vi "Configure Humidifiers.vi"(8 "error in":errorcluster, 10 "Humidifier":string="Med", 11 "Controller in":refnum<class "Controller.lvclass">) -> (0 "error out":errorcluster, 1 "TEC Handle":string, 2 "Vaisala Handle":string, 3 "Controller Out":refnum<class "Controller.lvclass">, 5 "MFC":string)   [LabVIEW 2014, in "Controller.lvlib" / "Controller.lvclass"]
uses:
  Controller.lvclass
  reusable/Session APIs/File Access/Config Data/Config Data.lvclass
  <vilib>/Utility/config.llb/NI_LVConfig.lvlib
  <vilib>/Utility/config.llb/Read Key (String).vi
  <vilib>/Utility/config.llb/Read Key (Double).vi
  reusable/Session APIs/CVT/CVT.lvclass
  <vilib>/Utility/config.llb/Read Key (Boolean).vi
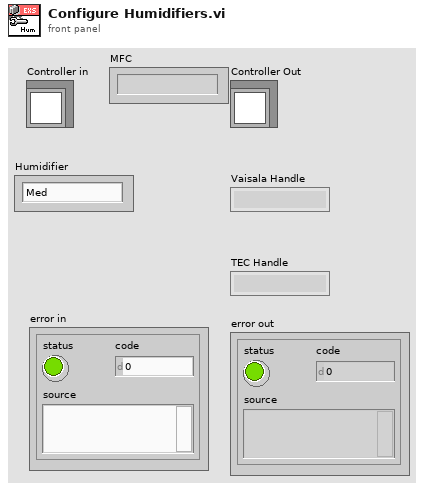
[diagram p1: front panel]
types:
  T1 = typedef "Session - Root.lvclass/Session Handle.ctl" = refnum<data-value>
  T2 = typedef "NI_LVConfig.lvlib/Config Data RefNum.ctl" = refnum<k1>
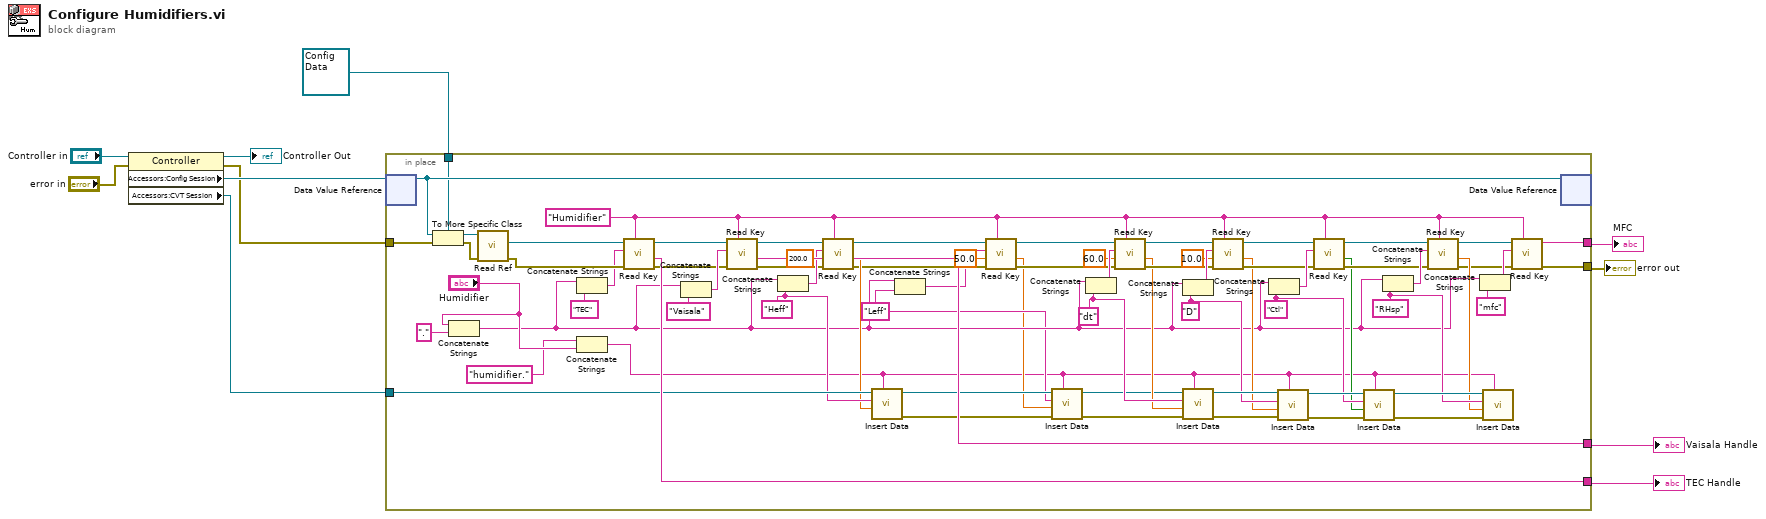
[diagram p0: block diagram]
diagram:
  n1 = property class="Controller"(reference="Controller in", error in="error in") -> (reference out=→"Controller Out":refnum<class "Controller.lvclass">, error out=w3:errorcluster, "Accessors:Config Session"=w7:T1, "Accessors:CVT Session"=w6:T1)
  n2 = in-place {
    in-place-border: refnum<class "Config Data.lvclass"> refnum ("Config Data in") -> [w81]
    in-place-border: [w79] -> w10
    in-place-border: [w78] -> w11
    in-place-border: w3 -> [w76]
    in-place-border: w6 -> [w75]
    in-place-border: [w31] -> w2
    in-place-border: [w29] -> w1
    w18 = "Leff" ("string")
    w39 = "RHsp" ("string")
    w43 = "Ctl" ("string")
    w47 = "D" ("string")
    w51 = "dt" ("string")
    w53 = "Heff" ("string")
    w21 = "Humidifier" ("section")
    n3 = in-place-dvr #1(w7) -> (w82:refnum<class "Session - Root.lvclass">)  [unwired: 1 out]
    n4 = To More Specific Class(target class=w81, reference=w82, error in=w76) -> (specific class reference=w77:refnum<class "Config Data.lvclass">, error out=w83:errorcluster)
    n5 = Concatenate Strings("Humidifier", "." ("string")) -> (w23:string)
    n6 = call "Read Ref.vi"("error in"=w83, "Config Data in"=w77) -> ("error out"=w74:errorcluster, "config data"=w80:T2)  [unwired: 7 in, 1 out]
    n7 = Concatenate Strings(w23, "TEC" ("string")) -> (w72:string)
    n8 = Concatenate Strings("humidifier.", "Humidifier") -> (w16:string)
    n9 = call-poly <vilib>:"Read Key.vi"("section"=w21, "error in (no error)"=w74, "key"=w72, "refnum"=w80) -> ("error out"=w58:errorcluster, "value"=w79:string, "refnum out"=w69:T2)  [unwired: 4 in, 1 out]
    n10 = Concatenate Strings(w23, "Vaisala" ("string")) -> (w70:string)
    n11 = call-poly <vilib>:"Read Key.vi"("section"=w21, "error in (no error)"=w58, "key"=w70, "refnum"=w69) -> ("error out"=w57:errorcluster, "value"=w78:string, "refnum out"=w68:T2)  [unwired: 4 in, 1 out]
    n12 = Concatenate Strings(w23, w53) -> (w67:string)
    n13 = call-poly <vilib>:"Read Key.vi"("section"=w21, "error in (no error)"=w57, "default value"=200.0, "key"=w67, "refnum"=w68) -> ("error out"=w25:errorcluster, "value"=w52:dbl, "refnum out"=w66:T2)  [unwired: 3 in, 1 out]
    n14 = call "Insert Data.vi"("Group"=w16, "Data"=w52, "tag"=w53, "CVT Session In"=w75) -> ("error out"=w27:errorcluster, "CVT Session Out"=w28:T1)  [unwired: 6 in]
    n15 = Concatenate Strings(w23, w18) -> (w22:string)
    n16 = call-poly <vilib>:"Read Key.vi"("section"=w21, "error in (no error)"=w25, "default value"=50.0, "key"=w22, "refnum"=w66) -> ("error out"=w24:errorcluster, "value"=w17:dbl, "refnum out"=w26:T2)  [unwired: 3 in, 1 out]
    n17 = call "Insert Data.vi"("Group"=w16, "error in"=w27, "Data"=w17, "tag"=w18, "CVT Session In"=w28) -> ("error out"=w20:errorcluster, "CVT Session Out"=w19:T1)  [unwired: 5 in]
    n18 = Concatenate Strings(w23, w51) -> (w65:string)
    n19 = call-poly <vilib>:"Read Key.vi"("section"=w21, "error in (no error)"=w24, "default value"=60.0, "key"=w65, "refnum"=w26) -> ("error out"=w56:errorcluster, "value"=w50:dbl, "refnum out"=w64:T2)  [unwired: 3 in, 1 out]
    n20 = Concatenate Strings(w23, w47) -> (w63:string)
    n21 = call "Insert Data.vi"("Group"=w16, "error in"=w20, "Data"=w50, "tag"=w51, "CVT Session In"=w19) -> ("error out"=w48:errorcluster, "CVT Session Out"=w49:T1)  [unwired: 5 in]
    n22 = call-poly <vilib>:"Read Key.vi"("section"=w21, "error in (no error)"=w56, "default value"=10.0, "key"=w63, "refnum"=w64) -> ("error out"=w55:errorcluster, "value"=w46:dbl, "refnum out"=w62:T2)  [unwired: 3 in, 1 out]
    n23 = Concatenate Strings(w23, w43) -> (w61:string)
    n24 = call "Insert Data.vi"("Group"=w16, "error in"=w48, "Data"=w46, "tag"=w47, "CVT Session In"=w49) -> ("error out"=w45:errorcluster, "CVT Session Out"=w44:T1)  [unwired: 5 in]
    n25 = call-poly <vilib>:"Read Key.vi"("section"=w21, "error in (no error)"=w55, "key"=w61, "refnum"=w62) -> ("error out"=w54:errorcluster, "value"=w42:bool, "refnum out"=w60:T2)  [unwired: 4 in, 1 out]
    n26 = call "Insert Data.vi"("Group"=w16, "error in"=w45, "Data"=w42, "tag"=w43, "CVT Session In"=w44) -> ("error out"=w40:errorcluster, "CVT Session Out"=w41:T1)  [unwired: 5 in]
    n27 = Concatenate Strings(w23, w39) -> (w59:string)
    n28 = call-poly <vilib>:"Read Key.vi"("section"=w21, "error in (no error)"=w54, "key"=w59, "refnum"=w60) -> ("error out"=w32:errorcluster, "value"=w38:dbl, "refnum out"=w30:T2)  [unwired: 4 in, 1 out]
    n29 = Concatenate Strings(w23, "mfc") -> (w33:string)
    n30 = call "Insert Data.vi"("Group"=w16, "error in"=w40, "Data"=w38, "tag"=w39, "CVT Session In"=w41) -> ()  [unwired: 5 in, 2 out]
    n31 = call-poly <vilib>:"Read Key.vi"("section"=w21, "error in (no error)"=w32, "key"=w33, "refnum"=w30) -> ("error out"=w31:errorcluster, "value"=w29:string)  [unwired: 4 in, 2 out]
    n32 = in-place-dvr #1(w82) -> ()  [unwired: 2 out]
  }
  "Vaisala Handle" <- w11
  "TEC Handle" <- w10
  "error out" <- w2
  "MFC" <- w1
